vi "AppendToFile.vi"(9 "File Path":string, 10 "File Name":string, 11 "Text to add":string) -> ()   [LabVIEW 2010]
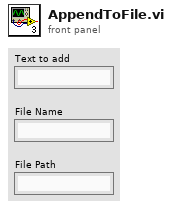
[diagram p1: front panel]
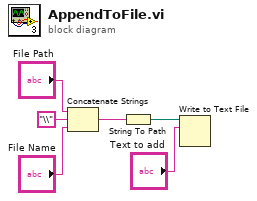
[diagram p0: block diagram]
diagram:
  n1 = Concatenate Strings("File Path", "\\" ("string"), "File Name") -> (w5:string)
  n2 = String To Path(string=w5) -> (path=w4:path)
  n3 = Write to Text File(file (use dialog)=w4, text="Text to add") -> ()  [unwired: 2 in, 3 out]
